vi "Main.vi"(11 "Module Admin":refnum<class "Delacor_lib_QMH_Module Admin.lvclass">) -> ()   [LabVIEW 2022 SP3, in "Acquire to AVI.lvlib"]
doc: "This template is based off of the Queued Message Handler design pattern and the Queued Message Handler project template that ships with LabVIEW.\n\nThe main difference is that the queue is private to this module and communication between modules is performed via Broadcast and Request events.\n\nRequest events are wrapped in public API methods and are handled in the Event Handling Loop (EHL) of this VI. Any module can register for Broadcast events sent by this module. The EHL generates messages based on user interface actions.\n\nThe Message Handling Loop (MHL) processes messages generated by the EHL, or by other messages. The messages are string values, so new messages can be added easily to the Message Cases case structure in the MHL. Each message cluster can also provide an optional value for Message Data, which is a variant that can be converted to whatever message-specific data is required.\n_____\nBased on DQMH Project Template 6.1.0.94."
uses:
  Acquire to AVI.lvlib
  <vilib>/Delacor/Delacor QMH/Libraries/Module Admin_class/Delacor_lib_QMH_Module Admin.lvclass
  Module Data--cluster.ctl
  <vilib>/Delacor/Delacor QMH/Libraries/Message Queue_class/Delacor_lib_QMH_Message Queue.lvclass/Delacor_lib_QMH_Message Queue.ctl
  Stop Argument--cluster.ctl
  <vilib>/Delacor/Delacor QMH/Libraries/Module Admin_class/Delacor_lib_QMH_Module Admin.lvclass/Delacor_lib_QMH_Module Admin.ctl
  Start acquire AVI Argument--cluster.ctl
  Stop acquire to AVI Argument--cluster.ctl
  <vilib>/Utility/miscctls.llb/LVPointTypeDef.ctl
  <vilib>/Delacor/Delacor QMH/Libraries/Message Queue_class/Delacor_lib_QMH_Enqueue Message (Single).vi
  <vilib>/Delacor/Delacor QMH/Libraries/Module Admin_class/Delacor_lib_QMH_Get External Launch.vi
  <vilib>/Utility/error.llb/Error Cluster From Error Code.vi
  <vilib>/ErrorRing/Error Ring.xnode
  <vilib>/Delacor/Delacor QMH/Libraries/Message Queue_class/Delacor_lib_QMH_Message Queue.lvclass
panel:
  out "time 2":i64
  out "num":i64
  out "time":i64
  out "new picture":picture
  out "Stopped butt":bool
  out "Image Out":T1(plugin-control)
  out "FPS":dbl
  out "appended path":path
  out "Gest":string="Gest1.png"
  out "Rec":bool
  in  "Start":bool
  in  "Stop (F)":bool
  out "error out":errorcluster
  out "Status":string
  in  "Simulate MHL Error":bool
  in  "Simulate EHL Error":bool
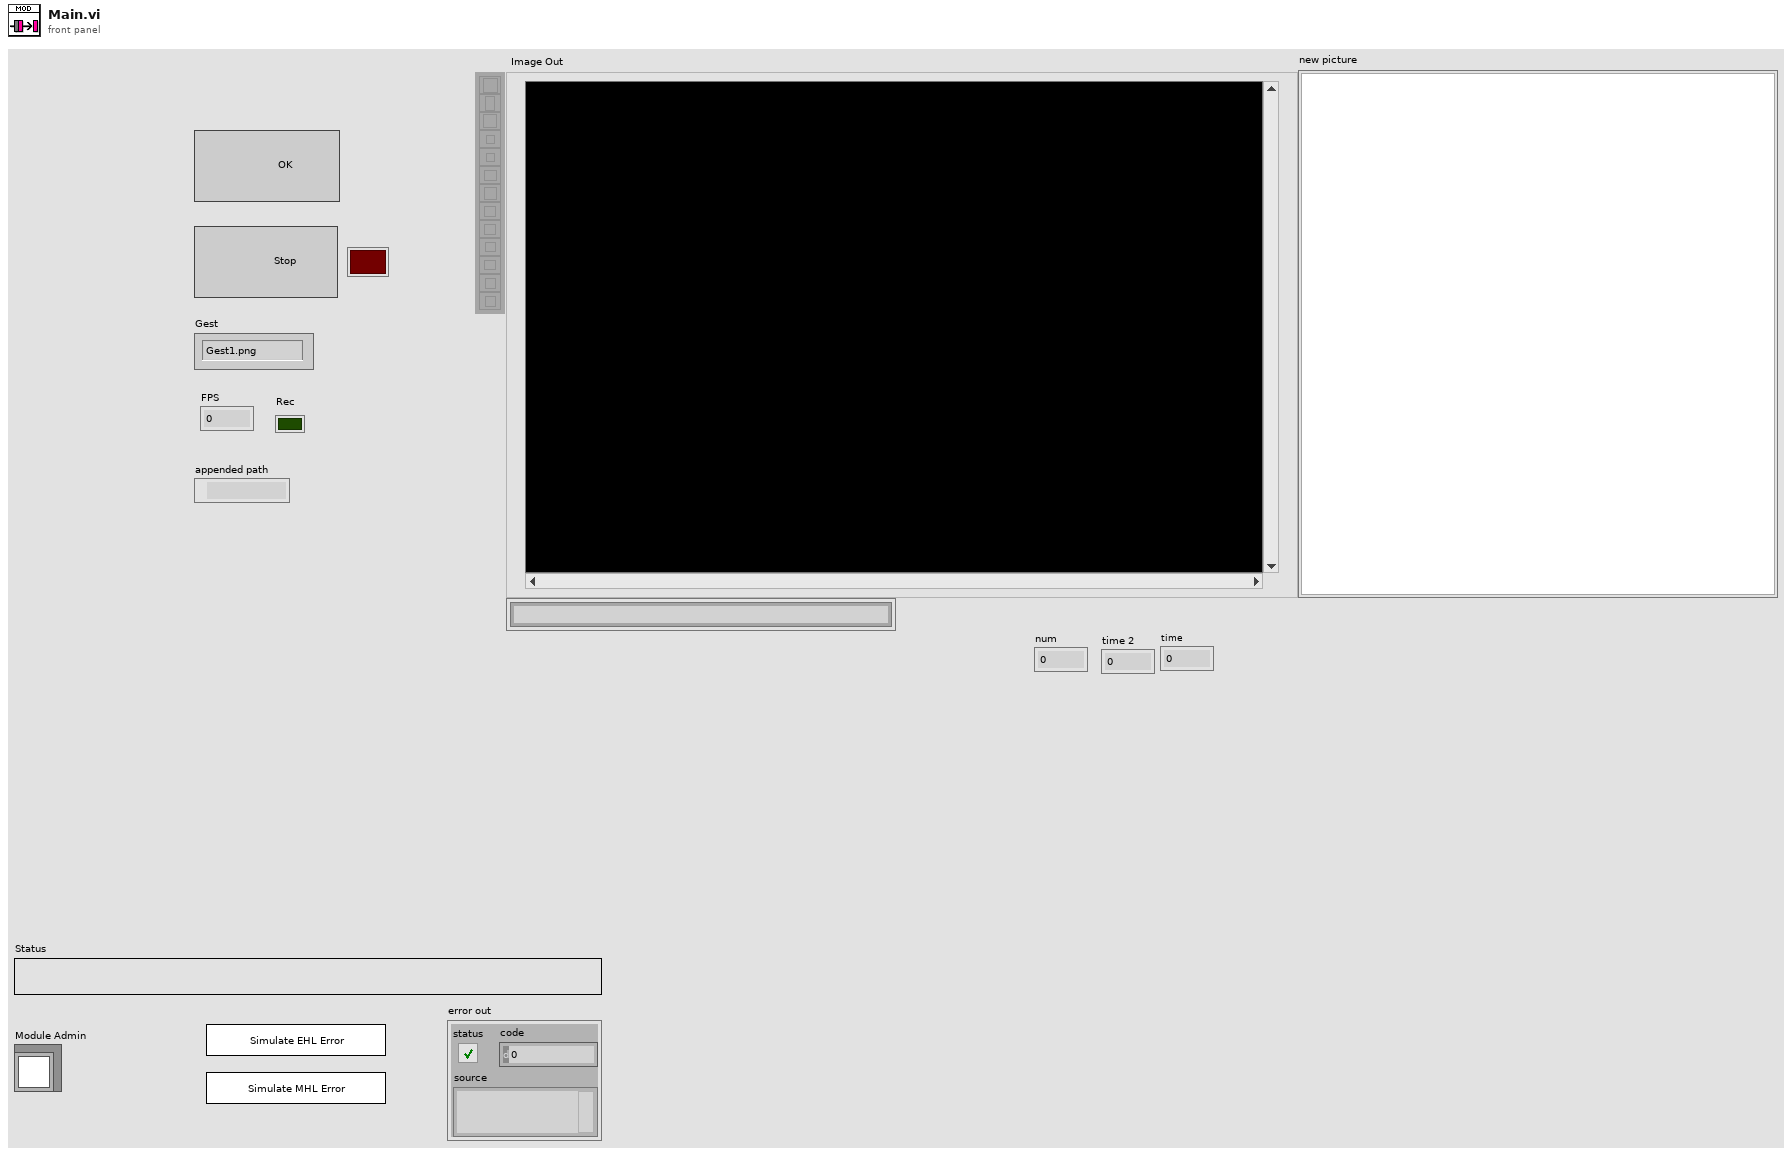
[diagram p1: front panel]
types:
  T1 = typedef "IMAQ Image.ctl" = refnum<image>
  T2 = typedef "Acquire to AVI.lvlib/Request Events--cluster.ctl" = cluster{"Stop Module":refnum<user-event>, "Show Panel":refnum<user-event>, "Hide Panel":refnum<user-event>, "Get Module Execution Status":refnum<user-event>, "Show Diagram":refnum<user-event>, "Acquire AVI":refnum<user-event>, "Start acquire AVI":refnum<user-event>, "Stop acquire to AVI":refnum<user-event>, "Start helper loop":refnum<user-event>, "Stop helper loop":refnum<user-event>}
  T3 = typedef "Acquire to AVI.lvlib/Module Data--cluster.ctl" = cluster{"Status":string}
  T4 = enum32{"invalid lock state", "Not Locked", "Locked (No Password)", "Password-protected"}
  T5 = typedef "Acquire to AVI.lvlib/Stop Argument--cluster.ctl" = cluster{"Origin":string, "Exit via Stop Module Req?":bool, "Wait for Module to stop?":bool}
  T6 = typedef "Acquire to AVI.lvlib/Start acquire AVI Argument--cluster.ctl" = cluster{"Boolean":bool}
  T7 = typedef "Acquire to AVI.lvlib/Stop acquire to AVI Argument--cluster.ctl" = cluster{"Boolean":bool}
  T8 = typedef "LVPointTypeDef.ctl" = cluster{"Horizontal":i16, "Vertical":i16}
  T9 = enum32{"Invalid", "Standard", "Closed", "Hidden", "Minimized", "Maximized"}
  T10 = cluster{"Global Rectangle":i32[], "Contours":cluster{"Contour Type":u32, "ROI Type":u32, "Points":i32[]}[]}
  T11 = typedef "imagedata.ctl" = cluster{"image type":i32, "image depth":i32, "image":u8[], "mask":u8[], "colors":u32[], "Rectangle":cluster{"left":i16, "top":i16, "right":i16, "bottom":i16}}
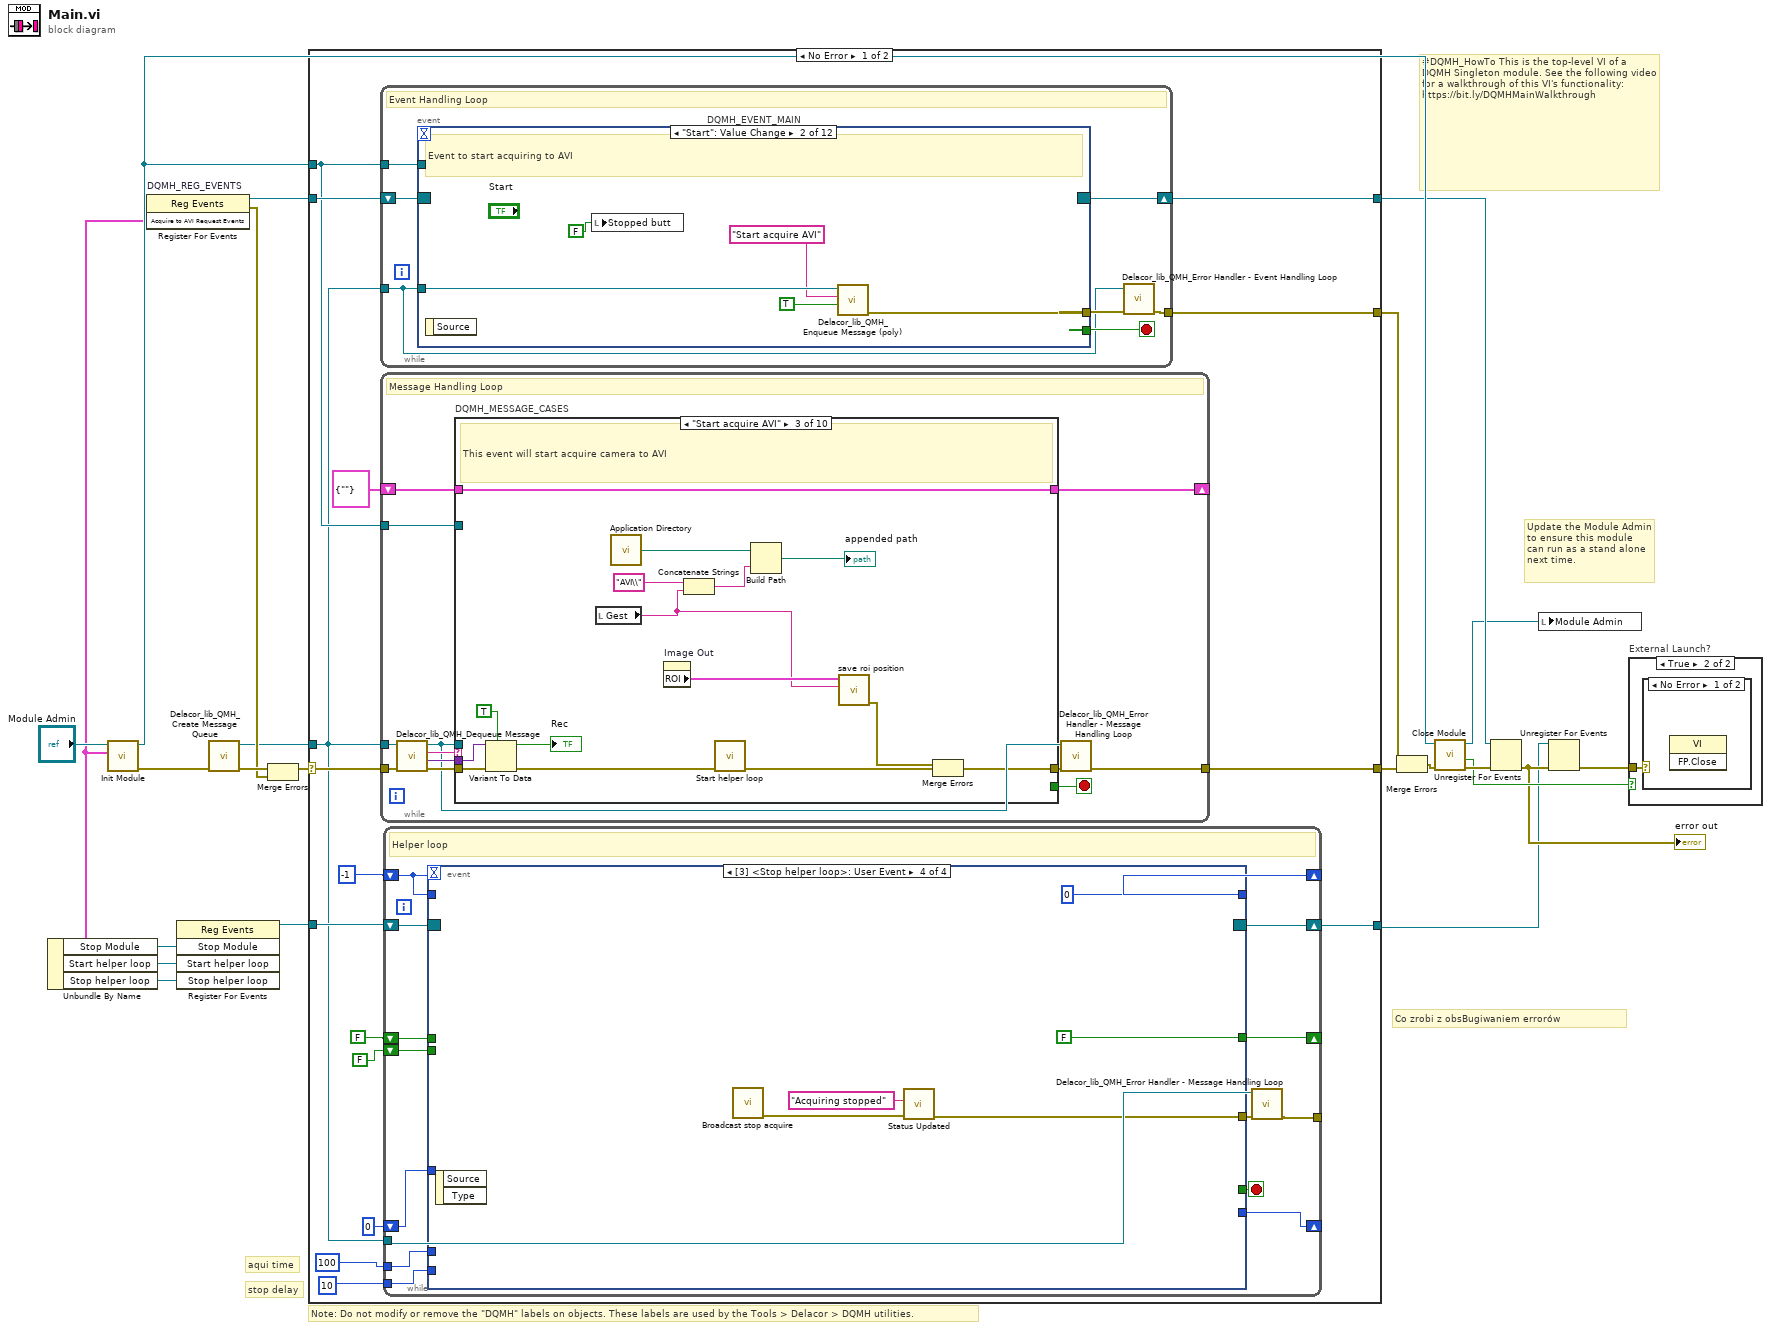
[diagram p0: block diagram]
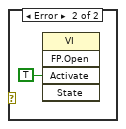
[diagram p3: hidden frame]
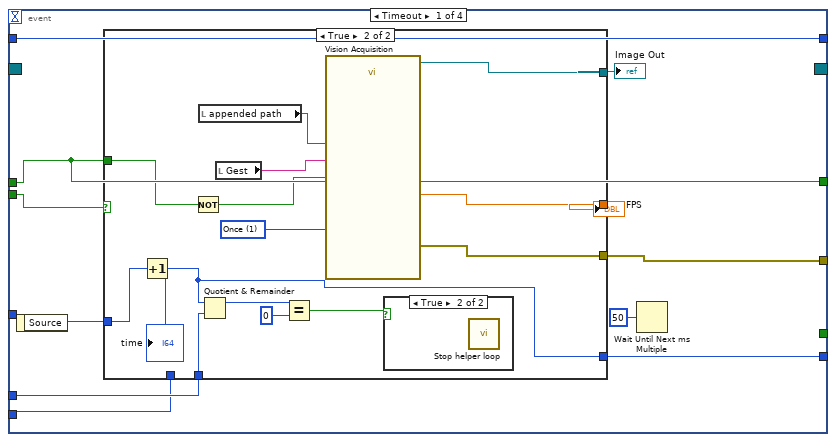
[diagram p4: hidden frame]
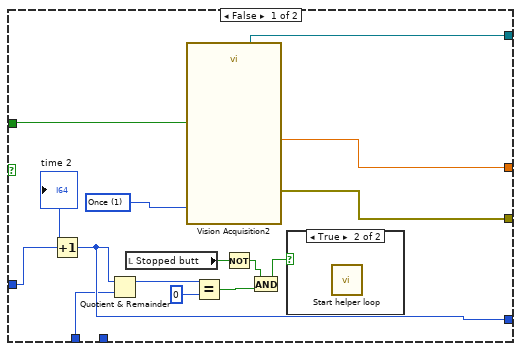
[diagram p5: hidden frame]
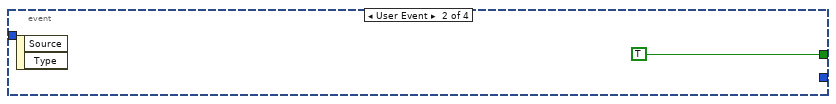
[diagram p8: hidden frame]
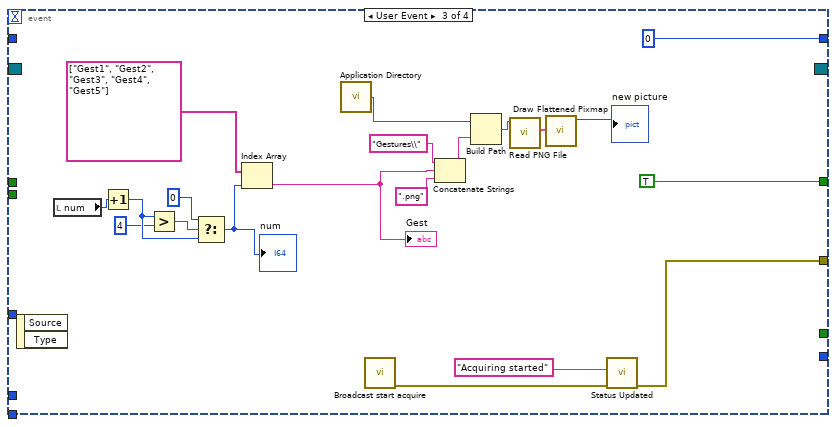
[diagram p9: hidden frame]
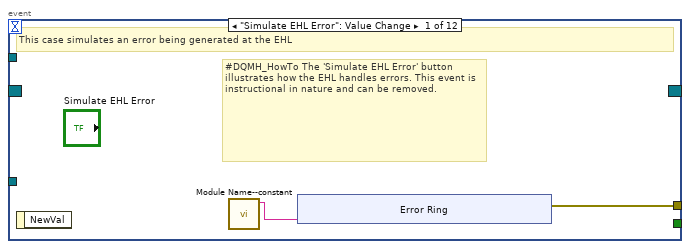
[diagram p10: hidden frame]
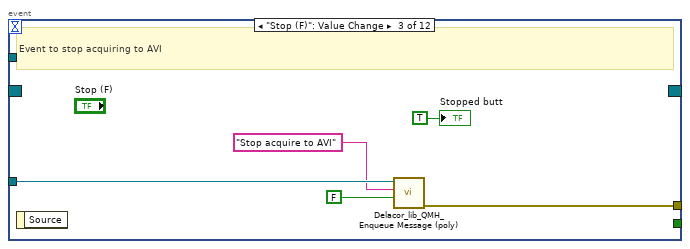
[diagram p11: hidden frame]
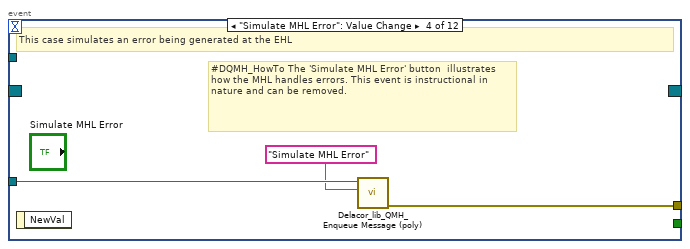
[diagram p12: hidden frame]
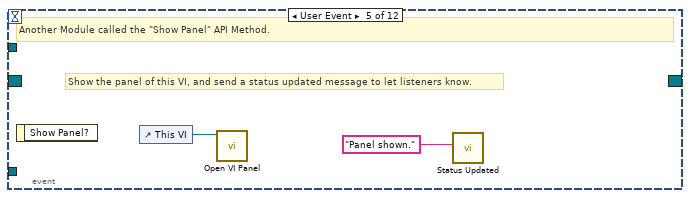
[diagram p13: hidden frame]
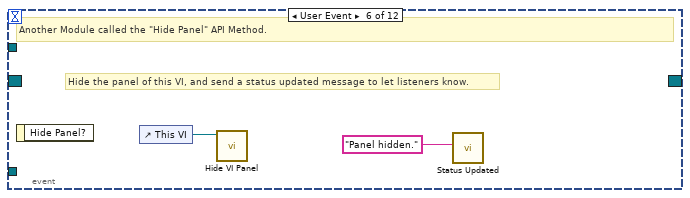
[diagram p14: hidden frame]
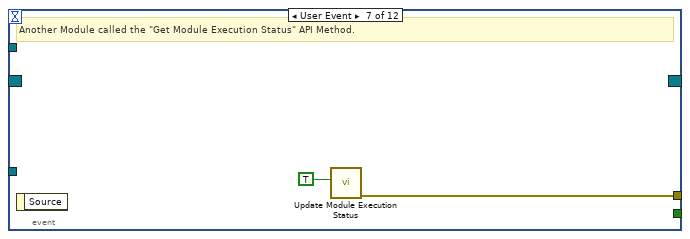
[diagram p15: hidden frame]
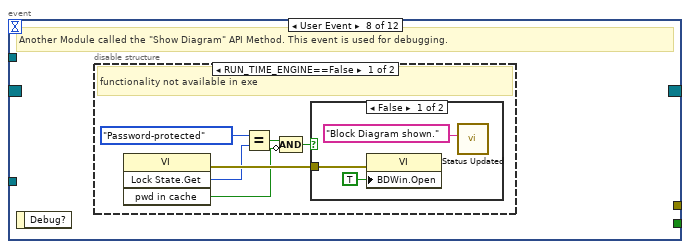
[diagram p16: hidden frame]
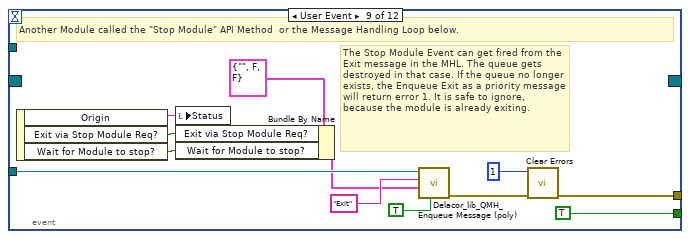
[diagram p19: hidden frame]
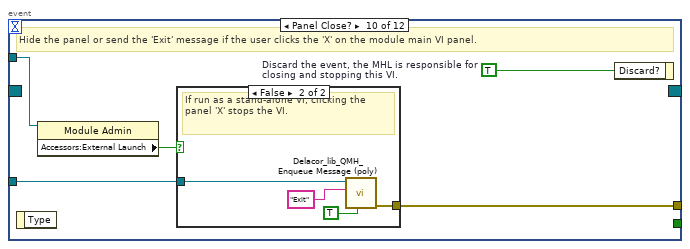
[diagram p20: hidden frame]
diagram:
  # "aqui time"
  # "stop delay"
  # "Co zrobi z obsBugiwaniem errorów"
  # "#DQMH_HowTo This is the top-level VI of a DQMH Singleton module. See the following video for a walkthrough of this VI's functionality: https://bit.ly/DQMHMainWalkthrough"
  # "Note: Do not modify or remove the \"DQMH\" labels on objects. These labels are used by the Tools > Delacor > DQMH utilities."
  # "Update the Module Admin to ensure this module can run as a stand alone next time."
  n1 = call "Init Module.vi"("Singleton Module Admin in"="Module Admin") -> ("error out"=w22:errorcluster, "Acquire to AVI Request Events"=w5:T2, "Singleton Module Admin out"=w15:refnum<class "Delacor_lib_QMH_Module Admin.lvclass">)  [unwired: 8 in]
  n2 = Unbundle By Name(w5) -> ("Stop Module"=w4:refnum<user-event>, "Start helper loop"=w3:refnum<user-event>, "Stop helper loop"=w2:refnum<user-event>)
  n3 = register-events "DQMH_REG_EVENTS"(w5) -> (reference out=w13:refnum<event-registration>, error out=w16:errorcluster)  [unwired: 2 in]
  n4 = register-events(w4, w3, w2) -> (reference out=w1:refnum<event-registration>)  [unwired: 2 in, 1 out]
  n5 = call <vilib>:"Delacor_lib_QMH_Create Message Queue.vi"("error in"=w22) -> ("error out"=w18:errorcluster, "Message Queue"=w12:refnum<class "Delacor_lib_QMH_Message Queue.lvclass">)  [unwired: 9 in]
  n6 = Merge Errors(w18, w16) -> (w17:errorcluster)
  n7 = case shown="No Error" w17 {
    selector: w17 -> [w37 w320]
    tunnel: [w39 w319] -> w23
    tunnel: [w36 w325] -> w14
    tunnel: w13 -> [w34 w325]
    tunnel: w12 -> [w27 w318]
    tunnel: [w38 _] -> w20
    tunnel: w15 -> [w33 w321]
    tunnel: w1 -> [w32 w317]
    tunnel: [w28 w317] -> w7
    frame No Error {
      n8 = while {
        tunnel: w27 -> [w120]
        shift-right: [w123] -> w36
        shift-left: w34 -> [w124]
        tunnel: [w125] -> w38
        tunnel: w33 -> [w121]
        stop <- w122 stop-if-true
        # "Event Handling Loop"
        n9 = event "DQMH_EVENT_MAIN" shown="[1] \"Start\": Value Change" {
          selector: w124 -> [_ _ _ _ _ _ _ _ _ _ _ _]
          dyn-events: [_ _ _ _ _ _ _ _ _ _ _ _] -> w123
          timeout: _ -> [_ _ _ _ _ _ _ _ _ _ _ _]
          tunnel: [_ _ _ _ _ _ _ _ TRUE ("Discard?") _ _ _] -> w122
          tunnel: w120 -> [_ w140 w144 w147 _ _ _ _ w171 w178 w191 w197]
          tunnel: [w128 w139 w142 w148 _ _ w154 _ w174 w180 w186 w192] -> w126
          tunnel: w121 -> [_ _ _ _ _ _ _ _ _ w177 _ _]
          event "Simulate EHL Error": Value Change {
            # "#DQMH_HowTo The 'Simulate EHL Error' button  illustrates how the EHL handles errors. This event is instructional in nature and can be removed."
            # "This case simulates an error being generated at the EHL"
            n10 = event-data() -> ()  [unwired: 1 in, 1 out]
            n11 = call "Module Name--constant.vi"() -> ("Module Name"=w127:string)  [unwired: 11 in]
            n12 = xnode "Error Ring"("parameter 0"=w127) -> ("error out"=w128:errorcluster)
          }
          event "Start": Value Change {
            # "Event to start acquiring to AVI"
            n13 = event-data() -> ()  [unwired: 1 in, 1 out]
            n14 = local write "Stopped butt"(FALSE ("Boolean")) -> ()
            n15 = call-poly <vilib>:"Delacor_lib_QMH_Enqueue Message (poly).vi"("Message Data"=TRUE, "Message"="Start acquire AVI", "Message Queue in"=w140) -> ("error out"=w139:errorcluster)  [unwired: 7 in, 1 out]
          }
          event "Stop (F)": Value Change {
            # "Event to stop acquiring to AVI"
            n16 = event-data() -> ()  [unwired: 1 in, 1 out]
            n17 = call-poly <vilib>:"Delacor_lib_QMH_Enqueue Message (poly).vi"("Message Data"=FALSE, "Message"="Stop acquire to AVI", "Message Queue in"=w144) -> ("error out"=w142:errorcluster)  [unwired: 7 in, 1 out]
            "Stopped butt" <- TRUE ("Boolean")
          }
          event "Simulate MHL Error": Value Change {
            # "#DQMH_HowTo The 'Simulate MHL Error' button  illustrates how the MHL handles errors. This event is instructional in nature and can be removed."
            # "This case simulates an error being generated at the EHL"
            n18 = event-data() -> ()  [unwired: 1 in, 1 out]
            n19 = call-poly <vilib>:"Delacor_lib_QMH_Enqueue Message (poly).vi"("Message"="Simulate MHL Error", "Message Queue in"=w147) -> ("error out"=w148:errorcluster)  [unwired: 8 in, 1 out]
          }
          event User Event {
            # "Show the panel of this VI, and send a status updated message to let listeners know."
            # "Another Module called the \"Show Panel\" API Method."
            n20 = event-data() -> ()  [unwired: 1 in, 1 out]
            n21 = control-ref of="This VI"() -> (w150:refnum<vi>)
            n22 = call "Open VI Panel.vi"("VI"=w150) -> ()  [unwired: 10 in, 1 out]
            n23 = call "Status Updated.vi"("Status"="Panel shown." ("format string")) -> ()  [unwired: 10 in, 1 out]
          }
          event User Event {
            # "Hide the panel of this VI, and send a status updated message to let listeners know."
            # "Another Module called the \"Hide Panel\" API Method."
            n24 = event-data() -> ()  [unwired: 1 in, 1 out]
            n25 = control-ref of="This VI"() -> (w152:refnum<vi>)
            n26 = call "Hide VI Panel.vi"("VI"=w152) -> ()  [unwired: 10 in, 1 out]
            n27 = call "Status Updated.vi"("Status"="Panel hidden." ("format string")) -> ()  [unwired: 10 in, 1 out]
          }
          event User Event {
            # "Another Module called the \"Get Module Execution Status\" API Method."
            n28 = event-data() -> ()  [unwired: 1 in, 1 out]
            n29 = call "Update Module Execution Status.vi"("Running?"=TRUE) -> ("error out"=w154:errorcluster)  [unwired: 10 in]
          }
          event User Event {
            # "Another Module called the \"Show Diagram\" API Method. This event is used for debugging."
            n30 = event-data() -> ()  [unwired: 1 in, 1 out]
            n31 = disable-structure shown="RUN_TIME_ENGINE==False" {
              frame condition #0 (active) {
                # "functionality not available in exe"
                n32 = invoke class="VI" method="Lock State.Get"() -> (error out=w160:errorcluster, "Get Lock State"=w159:T4, "pwd in cache"=w156:bool)  [unwired: 4 in, 1 out]
                n33 = Equal?(x=T4."Password-protected", y=w159) -> (x = y?=w157:bool)
                n34 = Compound Arithmetic op=AND(w157, invert w156) -> (w155:bool)
                n35 = case shown="False" w155 {
                  tunnel: w160 -> [w163 _]
                  frame False {
                    n36 = property class="VI"(error in=w163, "BDWin.Open"=TRUE ("Block Diagram Window:Open")) -> ()  [unwired: 1 in, 2 out]
                    n37 = call "Status Updated.vi"("Status"="Block Diagram shown." ("format string")) -> ()  [unwired: 10 in, 1 out]
                  }
                  frame True {
                    # "Password-protected VI, and the password is not in the cache. Do not show the diagram."
                  }
                }
              }
              frame condition #1 {
              }
            }
          }
          event User Event {
            # "The Stop Module Event can get fired from the Exit message in the MHL. The queue gets destroyed in that case. If the queue no longer exists, the Enqueue Exit as a priority message will return error 1. It is safe to ignore, because the module is already exiting."
            # "Another Module called the \"Stop Module\" API Method  or the Message Handling Loop below."
            n38 = event-data() -> ("Origin"=w170:string, "Exit via Stop Module Req?"=w166:bool, "Wait for Module to stop?"=w165:bool)  [unwired: 1 in]
            n39 = local write "Status"(w170) -> ()
            n40 = Bundle By Name(cluster=T5 {"Origin"="", "Exit via Stop Module Req?"=FALSE, "Wait for Module to stop?"=FALSE} ("Stop Argument"), "Exit via Stop Module Req?"=w166, "Wait for Module to stop?"=w165) -> (w164:T5)
            n41 = call-poly <vilib>:"Delacor_lib_QMH_Enqueue Message (poly).vi"("Priority Message? (F)"=TRUE, "Message Data"=w164, "Message"="Exit", "Message Queue in"=w171) -> ("error out"=w175:errorcluster)  [unwired: 6 in, 1 out]
            n42 = call <vilib>:"Clear Errors.vi"("error in (no error)"=w175, "specific error code to clear (0: all)"=1) -> ("error out"=w174:errorcluster)  [unwired: 4 in, 1 out]
          }
          event Panel Close? {
            w179 = TRUE  # Discard the event, the MHL is responsible for closing and stopping this VI.
            # "Hide the panel or send the 'Exit' message if the user clicks the 'X' on the module main VI panel."
            n43 = event-data() -> ()  [unwired: 1 in, 1 out]
            n44 = property class="Module Admin"(reference=w177) -> ("Accessors:External Launch"=w176:bool)  [unwired: 1 in, 2 out]
            n45 = case shown="False" w176 {
              tunnel: w178 -> [_ w184]
              tunnel: [_ w185] -> w180
              frame True {
                # "If externally launched, clicking the 'X' hides the panel, but doesn't close it."
                n46 = control-ref of="This VI"() -> (w181:refnum<vi>)
                n47 = call "Hide VI Panel.vi"("VI"=w181) -> ()  [unwired: 10 in, 1 out]
              }
              frame False {
                # "If run as a stand-alone VI, clicking the panel 'X' stops the VI."
                n48 = call-poly <vilib>:"Delacor_lib_QMH_Enqueue Message (poly).vi"("Priority Message? (F)"=TRUE, "Message"="Exit", "Message Queue in"=w184) -> ("error out"=w185:errorcluster)  [unwired: 7 in, 1 out]
              }
            }
            n49 = event-data("Discard?"=w179) -> ()  [unwired: 1 in, 1 out]
          }
          event User Event {
            # "Another Module called the \"Start acquire AVI\" API Method."
            n50 = event-data() -> ("Boolean"=w187:bool)  [unwired: 1 in]
            n51 = Bundle(cluster=T6 {"Boolean"=FALSE} ("Start acquire AVI Argument"), "Boolean"=w187) -> (w188:T6)
            n52 = call-poly <vilib>:"Delacor_lib_QMH_Enqueue Message (poly).vi"("Message Data"=w188, "Message"="Start acquire AVI", "Message Queue in"=w191) -> ("error out"=w186:errorcluster)  [unwired: 7 in, 1 out]
          }
          event User Event {
            # "Another Module called the \"Stop acquire to AVI\" API Method."
            n53 = event-data() -> ("Boolean"=w193:bool)  [unwired: 1 in]
            n54 = Bundle(cluster=T7 {"Boolean"=FALSE} ("Stop acquire to AVI Argument"), "Boolean"=w193) -> (w194:T7)
            n55 = call-poly <vilib>:"Delacor_lib_QMH_Enqueue Message (poly).vi"("Message Data"=w194, "Message"="Stop acquire to AVI", "Message Queue in"=w197) -> ("error out"=w192:errorcluster)  [unwired: 7 in, 1 out]
          }
        }
        n56 = call-dynamic "Delacor_lib_QMH_Error Handler - Event Handling Loop.vi"("error in"=w126, "Message Queue in"=w120) -> ("dup error in"=w125:errorcluster)  [unwired: 8 in, 1 out]
      }
      n57 = while {
        tunnel: w27 -> [w200]
        shift-right: [w204] -> _
        shift-left: T3 {"Status"=""} ("Data Cluster") -> [w205]
        tunnel: w37 -> [w208]
        tunnel: [w206] -> w39
        tunnel: w33 -> [w198]
        stop <- w203 stop-if-true
        # "Message Handling Loop"
        n58 = call-dynamic "Delacor_lib_QMH_Dequeue Message.vi"("error in"=w208, "Message Queue in"=w200) -> ("error out"=w207:errorcluster, "Message Data"=w201:variant, "Message"=w202:string, "Message Queue out"=w199:refnum<class "Delacor_lib_QMH_Message Queue.lvclass">)  [unwired: 6 in]
        n59 = case "DQMH_MESSAGE_CASES" shown="\"Start acquire AVI\"" w202 {
          selector: w202 -> [_ _ _ _ _ _ _ _ _ w304]
          tunnel: w199 -> [_ _ _ _ _ _ _ w274 w296 _]
          tunnel: w207 -> [w228 w232 w247 w254 w257 w259 w264 w281 w302 w306]
          tunnel: [w210 w232 w234 w248 w256 w259 w263 w277 w299 w307] -> w209
          tunnel: w205 -> [w218 w231 w246 w253 w255 w258 w261 w276 w295 w305]
          tunnel: [w217 w231 w246 w253 w255 w258 w261 w276 w295 w305] -> w204
          tunnel: [_ _ _ _ _ _ _ _ w294 _] -> w203
          tunnel: w201 -> [_ _ w245 w252 _ _ _ w275 w293 _]
          tunnel: w198 -> [w219 _ _ _ _ _ _ w273 w288 _]
          frame "Initialize" {
            w213 = "Initial Message" ("Initial Message")
            # "#CodeNeeded - Initialize the appearance of the front panel."
            # "#CodeNeeded - Initialize your state data here."
            # "Initialize - Any operation that needs to be done before the module can receive messages. Synchronize Caller Events.vi will inform Start Module.vi that the module has launched and is ready to receive messages. Module Did Init.vi will broadcast that the module initialized."
            n60 = call "Synchronize Caller Events.vi"("error in (no error)"=w228, "Singleton Module Admin in"=w219) -> ("error out"=w227:errorcluster, "Singleton Module Admin out"=w214:refnum<class "Delacor_lib_QMH_Module Admin.lvclass">)  [unwired: 8 in]
            n61 = property class="Module Admin"(reference=w214) -> ("Accessors:External Launch"=w223:bool)  [unwired: 1 in, 2 out]
            n62 = Select(t=T9."Hidden" ("State"), s=w223, f=T9."Standard" ("State")) -> (s? t:f=w220:T9)
            n63 = call "Module Name--constant.vi"() -> ("Module Name"=w215:string)  [unwired: 11 in]
            n64 = call "Module Name--constant.vi"() -> ("Module Name"=w226:string)  [unwired: 11 in]
            n65 = property class="VI"("Front Panel.Title"=w226) -> (reference out=w225:refnum<vi>, error out=w230:errorcluster)  [unwired: 2 in]
            n66 = call "Module Did Init.vi"("error in (no error)"=w227, "Initialized?"=TRUE, "Origin"=w215) -> ("error out"=w211:errorcluster)  [unwired: 8 in]
            n67 = invoke class="VI" method="FP.Open"(reference=w225, error in=w230, "State"=w220) -> (reference out=w224:refnum<vi>, error out=w229:errorcluster)  [unwired: 2 in, 3 out]
            n68 = Bundle By Name(cluster=w218, "Status"=w213) -> (w217:T3)
            n69 = call "Start helper loop.vi"("error in"=w211) -> ("error out"=w210:errorcluster)  [unwired: 10 in]
            n70 = invoke class="VI" method="FP.Center"(reference=w224, error in=w229) -> ()  [unwired: 1 in, 3 out]
            n71 = property on="Pane" class="Pane"("Origin"=T8 {"Horizontal"=0, "Vertical"=0}) -> ()  [unwired: 2 in, 2 out]
            "Status" <- w213
          }
          frame "---Module Specific---" {
            # "Separator -- The following cases handle messages specific to this Module."
          }
          frame "Start acquire AVI" {
            # "This event will start acquire camera to AVI"
            n72 = Variant To Data(error in=w247, type=TRUE, Variant=w245) -> (data=→"Rec":bool, error out=w242:errorcluster)
            n73 = local read "Gest"() -> (w236:string)
            n74 = call <vilib>:"Application Directory.vi"() -> ("Application Directory"=w241:path)
            n75 = property on="Image Out" class="ImageControl"() -> ("ROI"=w237:T10)  [unwired: 2 in, 2 out]
            n76 = Concatenate Strings("AVI\\", w236) -> (w239:string)
            n77 = call "Start helper loop.vi"("error in"=w242) -> ("error out"=w235:errorcluster)  [unwired: 10 in]
            n78 = Build Path(base path=w241, name or relative path=w239) -> (appended path=→"appended path":path)
            n79 = call "save roi position.vi"("Gest"=w236, "input cluster"=w237) -> ("error out"=w233:errorcluster)  [unwired: 9 in]
            n80 = Merge Errors(w233, w235) -> (w234:errorcluster)
          }
          frame "Stop acquire to AVI" {
            # "This event will stop acquiring from camera to AVI."
            n81 = Variant To Data(error in=w254, type=FALSE, Variant=w252) -> (data=w250:bool, error out=w249:errorcluster)
            n82 = local write "Rec"(w250) -> ()
            n83 = call "Stop helper loop.vi"("error in"=w249) -> ("error out"=w248:errorcluster)  [unwired: 10 in]
          }
          frame "---Copy This Frame---" {
            # "Duplicate this frame when creating new messages.  Change this comment in the duplicated frame to describe this message."
            n84 = Merge Errors(w257) -> (w256:errorcluster)
          }
          frame "---Exit and Error Handling---" {
            # "Separator - The following cases handle errors and exit messages."
          }
          frame "Simulate MHL Error" {
            # "#DQMH_HowTo The 'Simulate MHL Error' button  illustrates how the MHL handles errors. This event is instructional in nature and can be removed."
            # "Simulate an error occurring at the MHL"
            n85 = call "Module Name--constant.vi"() -> ("Module Name"=w260:string)  [unwired: 11 in]
            n86 = xnode "Error Ring"("parameter 0"=w260) -> ("error out"=w262:errorcluster)
            n87 = Merge Errors(w264, w262) -> (w263:errorcluster)
          }
          frame "Error" {
            # "#CodeRecommended - If you ever change the name of this \"Error\" message, you'll need to update the name in the Check Loop Error.vi as well."
            # "#CodeRecommended - If the module is running in standalone mode (External Launch = FALSE), this code will pop up an error dialog and call the 'Exit' message if an error occurs. Add more fine-grained error handling here."
            # "Error - Check the error message data and respond accordingly. This message is sent by the \"Error Handler\" VIs at the end of each loop in this application."
            n88 = property class="Module Admin"(reference=w273) -> ("Accessors:External Launch"=w272:bool)  [unwired: 1 in, 2 out]
            n89 = Variant To Data(error in=w281, type=errorcluster {"status"=FALSE, "code"=0, "source"=""} ("error constant"), Variant=w275) -> (data=w282:errorcluster, error out=w279:errorcluster)
            n90 = call "Error Reported.vi"("Error"=w282) -> ()  [unwired: 10 in, 1 out]
            n91 = case shown="False" w272 {
              tunnel: [w287 _] -> w278
              tunnel: w274 -> [w285 _]
              tunnel: w282 -> [w286 _]
              frame False {
                # "If the module is running standalone, then pop up an error dialog and call the \"Exit\" message."
                n92 = call <vilib>:"Simple Error Handler.vi"("error in (no error)"=w286) -> ()  [unwired: 4 in, 5 out]
                n93 = call-poly <vilib>:"Delacor_lib_QMH_Enqueue Message (poly).vi"("Priority Message? (F)"=TRUE, "Message"="Exit", "Message Queue in"=w285) -> ("error out"=w287:errorcluster)  [unwired: 7 in, 1 out]
              }
              frame True {
                # "If the module was launched externally, calling the Error Reported broadcast VI is the only action performed by the \"Error\" message. The module's caller can then process the error appropriately."
              }
            }
            n94 = Merge Errors(w279, w278) -> (w277:errorcluster)
            n95 = local write "error out"(w277) -> ()
          }
          frame "Exit" {
            w292 = 91  # 91: not all Exit messages will have an argument
            w294 = TRUE  # Stop the VI
            # "Release the message queue reference"
            # "#CodeNeeded - Add any required cleanup code here"
            # "Exit - Exit the application."
            n96 = Variant To Data(error in=w302, type=T5 {"Origin"="", "Exit via Stop Module Req?"=FALSE, "Wait for Module to stop?"=FALSE} ("Stop Argument"), Variant=w293) -> (data=w290:T5, error out=w298:errorcluster)
            n97 = call <vilib>:"Clear Errors.vi"("error in (no error)"=w298, "specific error code to clear (0: all)"=w292) -> ("error out"=w301:errorcluster)  [unwired: 4 in, 1 out]
            n98 = control-ref of="This VI"() -> (w289:refnum<vi>)
            n99 = call-dynamic "Delacor_lib_QMH_Release Message Queue.vi"("error in"=w301, "Message Queue"=w296) -> ("error out"=w300:errorcluster)  [unwired: 9 in]
            n100 = call "Handle Exit.vi"("Stop Argument"=w290, "Admin in"=w288, "VI reference"=w289) -> ("error out"=w297:errorcluster)  [unwired: 7 in, 1 out]
            n101 = Merge Errors(w300, w297) -> (w299:errorcluster)
          }
          frame Default {
            # "'Default' case only runs if there is a message that isn't defined in any of the other cases.  Output a programming error."
            n102 = call "Module Name--constant.vi"() -> ("Module Name"=w303:string)  [unwired: 11 in]
            n103 = xnode "Error Ring"("parameter 0"=w304, "parameter 1"=w303) -> ("error out"=w308:errorcluster)
            n104 = Merge Errors(w306, w308) -> (w307:errorcluster)
          }
        }
        n105 = call-dynamic "Delacor_lib_QMH_Error Handler - Message Handling Loop.vi"("error in"=w209, "Message Queue in"=w199) -> ("dup error in"=w206:errorcluster)  [unwired: 8 in, 1 out]
      }
      n106 = while {
        shift-right: [w51] -> w28
        shift-left: w32 -> [w54]
        shift-right: [w52] -> _
        shift-left: -1 -> [w53]
        shift-right: [w50] -> _
        shift-left: FALSE -> [w48]
        shift-left: FALSE -> [w49]
        tunnel: w27 -> [w46]
        tunnel: [w44] -> _
        tunnel: i64 100 -> [w43]
        shift-right: [w41] -> _
        shift-left: i64 0 -> [w42]
        tunnel: 10 -> [w40]
        stop <- w47 stop-if-true
        # "Helper loop"
        n107 = event shown="[3] <Stop helper loop>: User Event" {
          selector: w54 -> [_ _ _ _]
          dyn-events: [_ _ _ _] -> w51
          timeout: w53 -> [_ _ _ _]
          tunnel: w53 -> [w65 _ _ _]
          tunnel: [w65 _ 0 0] -> w52
          tunnel: [w61 _ TRUE FALSE] -> w50
          tunnel: [w64 _ w111 w115] -> w45
          tunnel: w49 -> [w62 _ _ _]
          tunnel: w48 -> [w61 _ _ _]
          tunnel: [_ TRUE _ _] -> w47
          tunnel: w43 -> [w58 _ _ _]
          tunnel: w42 -> [w59 _ _ _]
          tunnel: [w57 _ _ _] -> w41
          tunnel: w40 -> [w56 _ _ _]
          event Timeout {
            n108 = event-data() -> ()  [unwired: 1 in, 1 out]
            n109 = case shown="True" w62 {
              tunnel: w61 -> [w75 w93]
              tunnel: [w78 w90] -> w64
              tunnel: [w77 w87] -> w63
              tunnel: [w76 w86] -> w55
              tunnel: w59 -> [w70 w85]
              tunnel: w58 -> [_ w82]
              tunnel: [w72 w81] -> w57
              tunnel: w56 -> [w71 _]
              frame False {
                w79 = u32 1 items=["Off", "Once"] ("Balance White Auto")
                n110 = Increment(x=w70) -> (x+1=w72:i64)
                "time 2" <- w72
                n111 = Quotient & Remainder(x=w72, y=w71) -> (x-y*floor(x/y)=w74:i64)  [unwired: 1 out]
                n112 = local read "Stopped butt"() -> (w68:bool)
                n113 = call "Vision Acquisition2"("White Balance::Mode"=w79, "Stop (F)"=w75) -> ("Image Out"=w76:T1, "Frame Rate"=w77:dbl, "error out"=w78:errorcluster)  [unwired: 22 in, 1 out]
                n114 = Equal?(x=w74, y=i64 0) -> (x = y?=w67:bool)
                n115 = Not(x=w68) -> (.not. x?=w69:bool)
                n116 = And(x=w69, y=w67) -> (x .and. y?=w66:bool)
                n117 = case shown="True" w66 {
                  frame False {
                  }
                  frame True {
                    n118 = call "Start helper loop.vi"() -> ()  [unwired: 11 in, 1 out]
                  }
                }
              }
              frame True {
                w91 = u32 1 items=["Off", "Once"] ("Balance White Auto")
                n119 = Increment(x=w85) -> (x+1=w81:i64)
                "time" <- w81
                n120 = Not(x=w93) -> (.not. x?=w92:bool)
                n121 = local read "appended path"() -> (w88:path)
                n122 = Quotient & Remainder(x=w81, y=w82) -> (x-y*floor(x/y)=w84:i64)  [unwired: 1 out]
                n123 = local read "Gest"() -> (w89:string)
                n124 = Equal?(x=w84, y=i64 0) -> (x = y?=w80:bool)
                n125 = call "Vision Acquisition"("Image Logging Path"=w88, "Image Logging Prefix"=w89, "White Balance::Mode"=w91, "Stop (F)"=w92) -> ("Image Out"=w86:T1, "Frame Rate"=w87:dbl, "error out"=w90:errorcluster)  [unwired: 19 in, 2 out]
                n126 = case shown="True" w80 {
                  frame False {
                  }
                  frame True {
                    n127 = call "Stop helper loop.vi"() -> ()  [unwired: 11 in, 1 out]
                  }
                }
              }
            }
            "FPS" <- w63
            "Image Out" <- w55
            n128 = Wait Until Next ms Multiple(millisecond multiple=u32 50) -> ()  [unwired: 1 out]
          }
          event User Event {
            n129 = event-data() -> ()  [unwired: 1 in, 2 out]
          }
          event User Event {
            n130 = event-data() -> ()  [unwired: 1 in, 2 out]
            n131 = local read "num"() -> (w101:i64)
            n132 = Increment(x=w101) -> (x+1=w107:i64)
            n133 = Greater?(x=w107, y=i64 4) -> (0:w108:bool)
            n134 = Select(t=i64 0, s=w108, f=w107) -> (s? t:f=w109:i64)
            "num" <- w109
            n135 = Index Array(array=string[] ["Gest1", "Gest2", "Gest3", "Gest4", "Gest5"], index=w109) -> (element=w102:string)
            "Gest" <- w102
            n136 = call <vilib>:"Application Directory.vi"() -> ("Application Directory"=w96:path)
            n137 = call "Broadcast start acquire.vi"() -> ("error out"=w112:errorcluster)  [unwired: 11 in]
            n138 = Concatenate Strings("Gestures\\", w102, ".png" ("string")) -> (w103:string)
            n139 = Build Path(base path=w96, name or relative path=w103) -> (appended path=w105:path)
            n140 = call <vilib>:"Read PNG File.vi"("path to PNG file"=w105) -> ("image data"=w106:T11)  [unwired: 8 in, 2 out]
            n141 = call <vilib>:"Draw Flattened Pixmap.vi"("image data"=w106) -> ("new picture"=→"new picture":picture)  [unwired: 8 in]
            n142 = call "Status Updated.vi"("error in (no error)"=w112, "Status"="Acquiring started") -> ("error out"=w111:errorcluster)  [unwired: 9 in]
          }
          event User Event {
            n143 = event-data() -> ()  [unwired: 1 in, 2 out]
            n144 = call "Broadcast stop acquire.vi"() -> ("error out"=w117:errorcluster)  [unwired: 11 in]
            n145 = call "Status Updated.vi"("error in (no error)"=w117, "Status"="Acquiring stopped") -> ("error out"=w115:errorcluster)  [unwired: 9 in]
          }
        }
        n146 = call-dynamic "Delacor_lib_QMH_Error Handler - Message Handling Loop.vi"("error in"=w45, "Message Queue in"=w46) -> ("dup error in"=w44:errorcluster)  [unwired: 8 in, 1 out]
      }
    }
    frame Error {
      # "Synchronize Caller Events.vi will inform Start Module.vi that the module has launched and will let the code calling Start Module.vi register for broadcasts and would permit the caller receive the broadcast that an error occurred at launch time."
      n147 = call-dynamic "Delacor_lib_QMH_Release Message Queue.vi"("error in"=w320, "Message Queue"=w318) -> ("error out"=w319:errorcluster)  [unwired: 9 in]
      n148 = call "Synchronize Caller Events.vi"("Singleton Module Admin in"=w321) -> ("error out"=w326:errorcluster)  [unwired: 9 in, 1 out]
      n149 = call "Module Name--constant.vi"() -> ("Module Name"=w324:string)  [unwired: 11 in]
      n150 = Format Into String(format string="An error occurred during initialization. %s is no longer running.", w324) -> (resulting string=w322:string)  [unwired: 2 in, 1 out]
      n151 = Merge Errors(w319, w326) -> (w327:errorcluster)
      n152 = call "Error Reported.vi"("Additional Information"=w322, "Error"=w327) -> ()  [unwired: 9 in, 1 out]
    }
  }
  n153 = Merge Errors(w20, w23) -> (w19:errorcluster)
  n154 = call "Close Module.vi"("error in (no error)"=w19, "Module Admin in"=w15) -> ("error out"=w21:errorcluster, "External Launch"=w9:bool, "Module Admin out"=w10:refnum<class "Delacor_lib_QMH_Module Admin.lvclass">)  [unwired: 7 in]
  n155 = Unregister For Events(event registration refnum=w14, error in=w21) -> (error out=w8:errorcluster)
  "error out" <- w8
  n156 = local write "Module Admin"(w10) -> ()
  n157 = Unregister For Events(event registration refnum=w7, error in=w8) -> (error out=w6:errorcluster)
  n158 = case "External Launch?" shown="True" w9 {
    tunnel: w6 -> [_ w328]
    frame False {
    }
    frame True {
      n159 = case shown="No Error" w328 {
        frame No Error {
          n160 = invoke class="VI" method="FP.Close"() -> ()  [unwired: 3 in, 3 out]
        }
        frame Error {
          n161 = invoke class="VI" method="FP.Open"("Activate"=TRUE ("Activate?")) -> ()  [unwired: 4 in, 5 out]
        }
      }
    }
  }
